vi "Caclulate Zero Crossing Point.vi"(8 "zero crossing point":bool, 10 "x[n-1]":fxp<+/-,16,2>, 11 "x[n]":fxp<+/-,16,2>) -> (0 "data valid":bool, 2 "zero crossing point":fxp<+/-,16,2>)   [LabVIEW 2011]
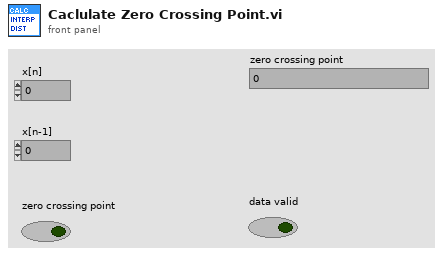
[diagram p1: front panel]
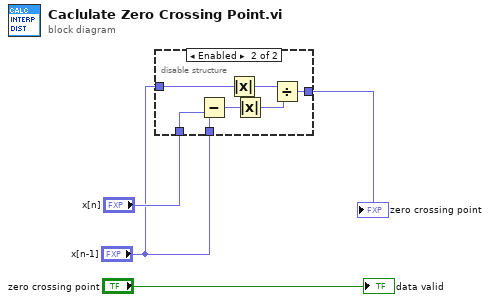
[diagram p0: block diagram]
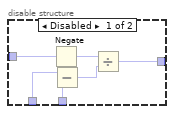
[diagram p2: hidden frame]
diagram:
  n1 = disable-structure shown="Enabled" {
    disable-tunnel: "x[n-1]" -> [w9 w13]
    disable-tunnel: "x[n]" -> [w8 w17]
    disable-tunnel: "x[n-1]" -> [w7 w16]
    disable-tunnel: [w5 w14] -> w2
    frame Disabled {
      n2 = Negate(x=w9) -> (-x=w10:fxp<+/-,17,3>)
      n3 = Subtract(x=w8, y=w7) -> (x-y=w6:fxp<+/-,17,3>)
      n4 = Divide(x=w10, y=w6) -> (x/y=w5:fxp<+/-,16,2>)
    }
    frame Enabled {
      n5 = Subtract(x=w16, y=w17) -> (x-y=w15:fxp<+/-,17,3>)
      n6 = Absolute Value(x=w13) -> (abs(x)=w11:fxp<+,16,2>)
      n7 = Absolute Value(x=w15) -> (abs(x)=w12:fxp<+,16,2>)
      n8 = Divide(x=w11, y=w12) -> (x/y=w14:fxp<+/-,16,2>)
    }
  }
  "zero crossing point" <- w2
  "data valid" <- "zero crossing point"
